vi "Autonomous_Parse.vi"(0 "File Path":path=path "C:/Users/theST/Desktop/Autonomous/Test.txt", 11 "error in":errorcluster) -> (1 "Name of Play":string, 2 "file text":string, 3 "DS Message":string, 4 "Number of Commands":i32, 6 "Subsystems":string[](array[string]), 8 "Commands":string[](array[string]), 10 "Inputs":string[][](array[string]), 15 "errror out":errorcluster)   [LabVIEW 2020]
uses:
  <vilib>/Utility/file.llb/Read Delimited Spreadsheet (string).vi
panel:
  out "Lines":string[](array[string])
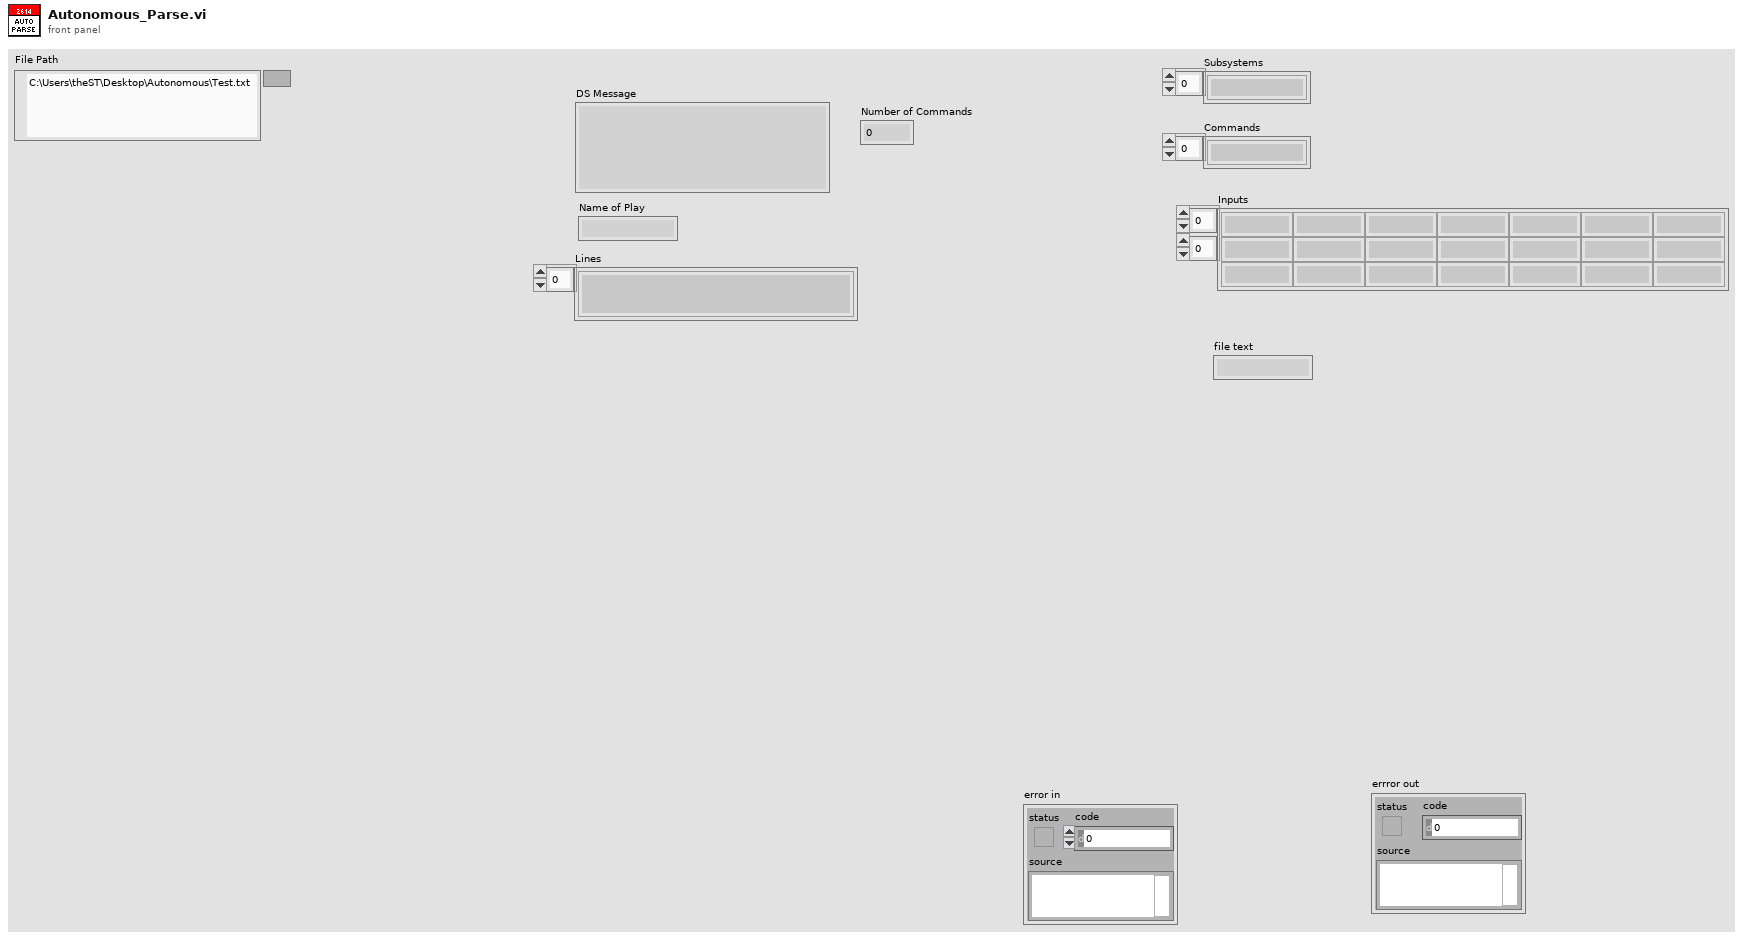
[diagram p1: front panel]
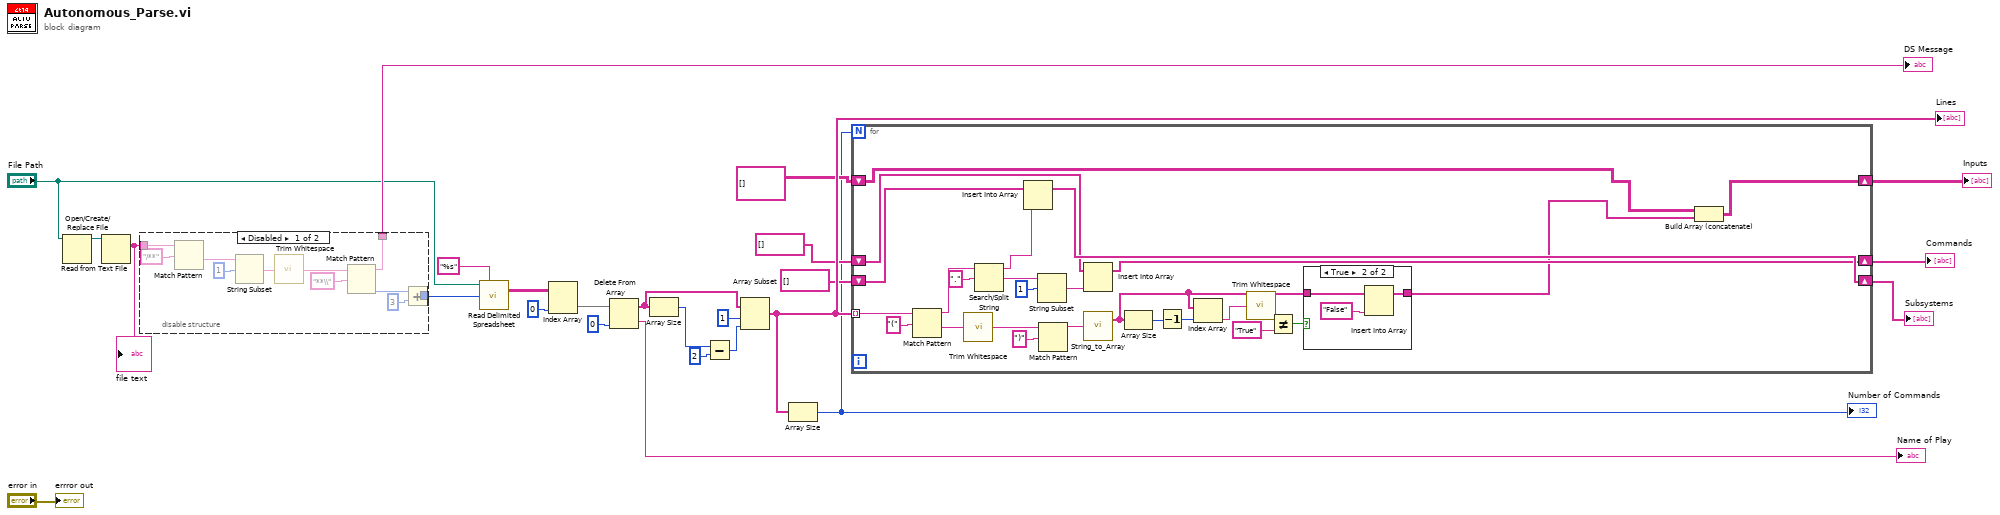
[diagram p0: block diagram]
diagram:
  n1 = Open/Create/Replace File(file path (use dialog)="File Path") -> (refnum out=w25:refnum<file>)  [unwired: 5 in, 2 out]
  n2 = Read from Text File(file (use dialog)=w25) -> (text=w8:string)  [unwired: 3 in, 3 out]
  "file text" <- w8
  n3 = disable-structure shown="Disabled" {
    disable-tunnel: [w36 _] -> w24
    disable-tunnel: [w35 _] -> w12
    disable-tunnel: w8 -> [w34 _]
    frame Disabled {
      n4 = Match Pattern(string=w34, regular expression="/**") -> (after substring=w32:string)  [unwired: 1 in, 3 out]
      n5 = String Subset(string=w32, offset (0)=1) -> (substring=w29:string)  [unwired: 1 in]
      n6 = call <vilib>:"Trim Whitespace.vi"("string"=w29) -> ("trimmed string"=w28:string)  [unwired: 1 in]
      n7 = Match Pattern(string=w28, regular expression="**\\") -> (before substring=w36:string, offset past match=w27:i32)  [unwired: 1 in, 2 out]
      n8 = Add(x=w27, y=3) -> (x+y=w35:i32)
    }
    frame Enabled {
    }
  }
  "DS Message" <- w24
  n9 = call-poly <vilib>:"Read Delimited Spreadsheet.vi"("file path (dialog if empty)"="File Path", "format (%s)"="%s", "start of read offset (chars.:0)"=w12) -> ("all rows"=w14:string[][])  [unwired: 7 in, 5 out]
  n10 = Index Array(array=w14, index (col)=0 ("disabled index (col)")) -> (element=w18:string[])  [unwired: 1 in]
  n11 = Delete From Array(array=w18, index=0) -> (deleted portion=→"Name of Play":string, array with subset deleted=w19:string[])  [unwired: 1 in]
  n12 = Array Size(array=w19) -> (size(s)=w22:i32)
  n13 = Subtract(x=w22, y=2) -> (x-y=w21:i32)
  n14 = Array Subset(array=w19, index=1, length=w21) -> (w11:string[])
  "Lines" <- w11
  n15 = Array Size(array=w11) -> (size(s)=w2:i32)
  "Number of Commands" <- w2
  n16 = for {
    N: w2 -> [_]
    tunnel: w11 -> [w59] mode=indexing
    shift-right: [w41] -> w1
    shift-left: string[][] [] ("appended array") -> [w43]
    shift-right: [w56] -> w10
    shift-left: string[] [] -> [w54]
    shift-right: [w55] -> w3
    shift-left: string[] [] -> [w53]
    n17 = Match Pattern(string=w59, regular expression="(") -> (before substring=w51:string, after substring=w62:string)  [unwired: 1 in, 2 out]
    n18 = call <vilib>:"Trim Whitespace.vi"("string"=w62) -> ("trimmed string"=w60:string)  [unwired: 1 in]
    n19 = Search/Split String(string=w51, search string/char (-)=".") -> (substring before match=w50:string, match + rest of string=w48:string)  [unwired: 1 in, 1 out]
    n20 = Insert Into Array(array=w54, new element=w50) -> (w56:string[])  [unwired: 1 in]
    n21 = String Subset(string=w48, offset (0)=1) -> (substring=w40:string)  [unwired: 1 in]
    n22 = Match Pattern(string=w60, regular expression=")") -> (before substring=w57:string)  [unwired: 1 in, 3 out]
    n23 = Insert Into Array(array=w53, new element=w40) -> (w55:string[])  [unwired: 1 in]
    n24 = call "String_to_Array.vi"("Input String"=w57) -> ("Array of Strings"=w45:string[])  [unwired: 1 out]
    n25 = Array Size(array=w45) -> (size(s)=w47:i32)
    n26 = Decrement(x=w47) -> (x-1=w46:i32)
    n27 = Index Array(array=w45, index=w46) -> (element=w38:string)
    n28 = call <vilib>:"Trim Whitespace.vi"("string"=w38) -> ("trimmed string"=w37:string)  [unwired: 1 in]
    n29 = Not Equal?(x=w37, y="True") -> (x != y?=w44:bool)
    n30 = case shown="True" w44 {
      tunnel: w45 -> [w63 w66]
      tunnel: [w63 w64] -> w42
      frame False {
      }
      frame True {
        n31 = Insert Into Array(array=w66, new element="False" ("new element/subarray")) -> (w64:string[])  [unwired: 1 in]
      }
    }
    n32 = Build Array (concatenate)(w43, w42) -> (w41:string[][])
  }
  "Subsystems" <- w10
  "Inputs" <- w1
  "Commands" <- w3
  "errror out" <- "error in"
